vi "LED Color - Copy.vi"(6 "Strings[4]":string, 8 "error in (no error)":errorcluster, 9 "T: F:Yellow; T:Red\nF: F:Yellow; T:Green":bool, 10 "Result":bool, 11 "Boolean Ref":refnum<vi>) -> (0 "error out":errorcluster)   [LabVIEW 2021]
panel:
  out "Array":string[](array[string])
  in  "Boolean 2":bool
  out "Boolean":bool
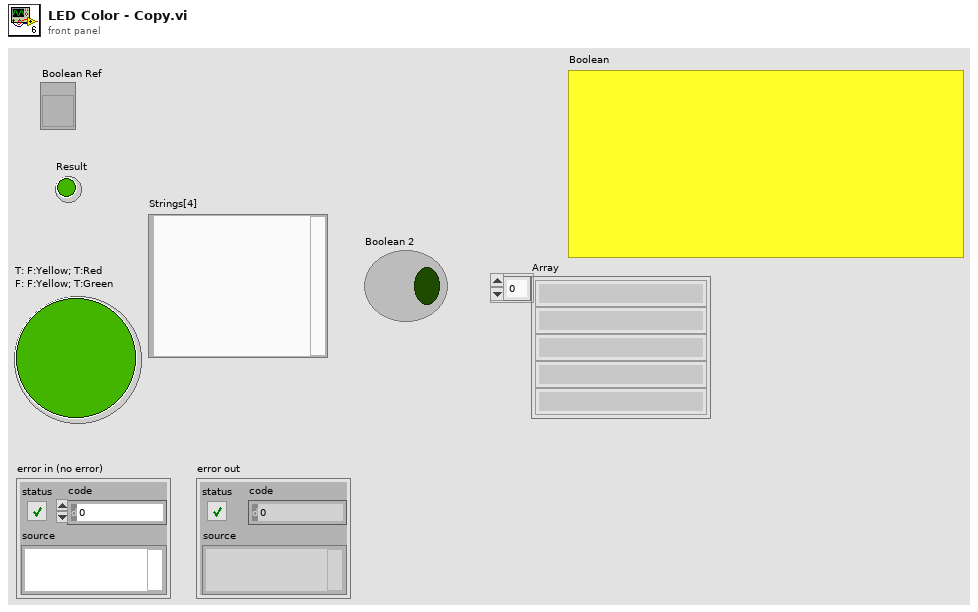
[diagram p1: front panel]
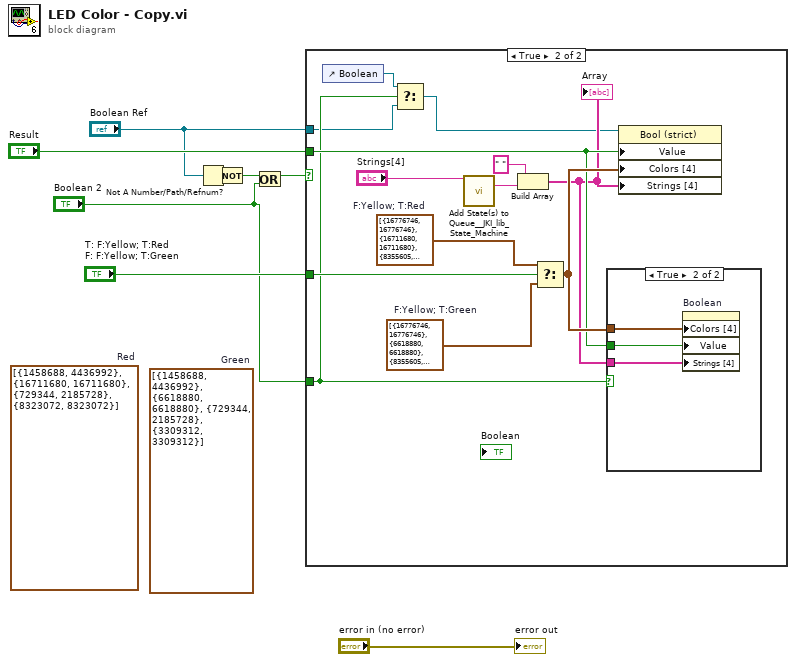
[diagram p0: block diagram]
diagram:
  (unwired) cluster{u32, u32}[] [{1458688, 4436992}, {6618880, 6618880}, {729344, 2185728}, {3309312, 3309312}]  # Green
  (unwired) cluster{u32, u32}[] [{1458688, 4436992}, {16711680, 16711680}, {729344, 2185728}, {8323072, 8323072}]  # Red
  n1 = Not A Number/Path/Refnum?(number/path/refnum="Boolean Ref") -> (NaN/Path/Refnum?=w5:bool)
  n2 = Not(x=w5) -> (.not. x?=w4:bool)
  n3 = Or(x=w4, y="Boolean 2") -> (x .or. y?=w3:bool)
  n4 = case shown="True" w3 {
    tunnel: "T: F:Yellow; T:Red\nF: F:Yellow; T:Green" -> [_ w21]
    tunnel: "Result" -> [_ w16]
    tunnel: "Boolean Ref" -> [_ w10]
    tunnel: "Boolean 2" -> [_ w12]
    frame False {
    }
    frame True {
      w20 = cluster{u32, u32}[] [{16776746, 16776746}, {16711680, 16711680}, {8355605, 8355605}, {8323072, 8323072}]  # F:Yellow; T:Red
      w19 = cluster{u32, u32}[] [{16776746, 16776746}, {6618880, 6618880}, {8355605, 8355605}, {3309312, 3309312}]  # F:Yellow; T:Green
      n5 = control-ref of="Boolean"() -> (w11:refnum<vi>)
      n6 = Select(t=w11, s=w12, f=w10) -> (s? t:f=w9:refnum<vi>)
      n7 = call <vilib>:"Add State(s) to Queue__JKI_lib_State_Machine.vi"("State(s) in Front (\"\")"="Strings[4]") -> ("States Out"=w15:string)  [unwired: 14 in]
      n8 = Build Array(" " ("element"), w15) -> (w14:string[])
      "Array" <- w14
      n9 = Select(t=w20, s=w21, f=w19) -> (s? t:f=w18:cluster{u32, u32}[])
      n10 = case shown="True" w12 {
        tunnel: w18 -> [_ w24]
        tunnel: w16 -> [_ w23]
        tunnel: w14 -> [_ w22]
        frame False {
        }
        frame True {
          n11 = property on="Boolean" class="Bool (strict)"("Colors [4]"=w24, "Value"=w23, "Strings [4]"=w22) -> ()  [unwired: 2 in, 2 out]
        }
      }
      n12 = property class="Bool (strict)"(reference=w9, "Value"=w16, "Colors [4]"=w18, "Strings [4]"=w14) -> ()  [unwired: 1 in, 2 out]
    }
  }
  "error out" <- "error in (no error)"
